vi "Test SSH API.vi"() -> ()   [LabVIEW 2017]
doc: "SSH API Tester."
uses:
  Response Configuration.ctl
  Expected Response String Config.ctl
  Search Start Point.ctl
  Connection Info.ctl
  <vilib>/Utility/config.llb/Write Key (String).vi
  <vilib>/Utility/config.llb/Write Key (I32).vi
  <vilib>/Utility/config.llb/Read Key (String).vi
  <vilib>/Utility/config.llb/Read Key (I32).vi
  SSH.lvlib
  <vilib>/Utility/config.llb/NI_LVConfig.lvlib
panel:
  in  "Load Config":bool
  in  "Save Config":bool
  in  "Write Response Configuration":T1
  in  "password":string
  in  "username":string
  in  "port":i32
  out "Response":string
  in  "Connection Name":string
  in  "host IP":string
  in  "Command":string
  in  "Write Command":bool
  in  "Run as Singleton?":bool
  in  "Show Block Diagram":bool
  in  "Refresh Modules":bool
  out "Active Modules":string[](array[string])
  in  "Stop Module":bool
  in  "Select Module":i32(ring)=-1 caption="Select Module\nTo send Request to" items=["All"=-1]
  in  "Run New Module":bool
  in  "Hide Module Panel":bool
  in  "Show Module Panel":bool
  out "Status":string
  # "This VI tests the API for the Module."
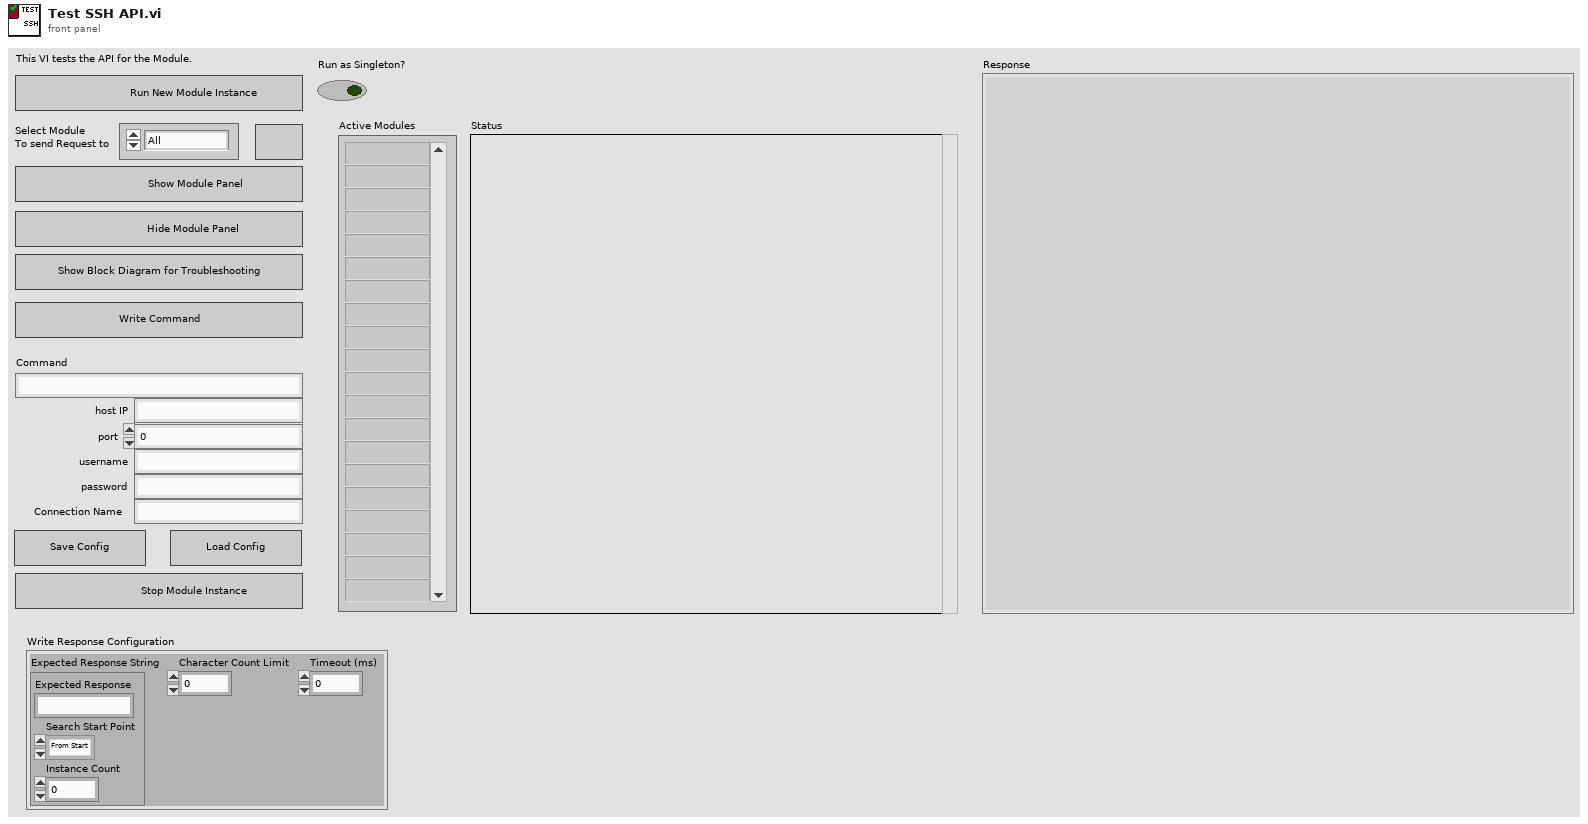
[diagram p1: front panel]
types:
  T1 = typedef "SSH.lvlib/Response Configuration.ctl" = cluster{"Expected Response String":T2, "Character Count Limit":i32, "Timeout (ms)":i32}
  T2 = typedef "SSH.lvlib/Expected Response String Config.ctl" = cluster{"Expected Response":string, "Search Start Point":T3, "Instance Count":i32}
  T3 = typedef "SSH.lvlib/Search Start Point.ctl" = enum16{"From Start", "From End"}
  T4 = typedef "SSH.lvlib/Broadcast Events--cluster.ctl" = cluster{"Module Did Init":refnum<user-event>, "Status Updated":refnum<user-event>, "Error Reported":refnum<user-event>, "Module Did Stop":refnum<user-event>, "Update Module Execution Status":refnum<user-event>}
  T5 = typedef "SSH.lvlib/Connection Info.ctl" = cluster{"host IP":string, "port":i32, "username":string, "password":string, "Connection Name":string}
  T6 = typedef "SSH.lvlib/Write Command (Reply Payload)--cluster.ctl" = cluster{"Write Command_error":errorcluster, "Return String Payload":string}
  T7 = typedef "NI_LVConfig.lvlib/Config Data RefNum.ctl" = refnum<k1>
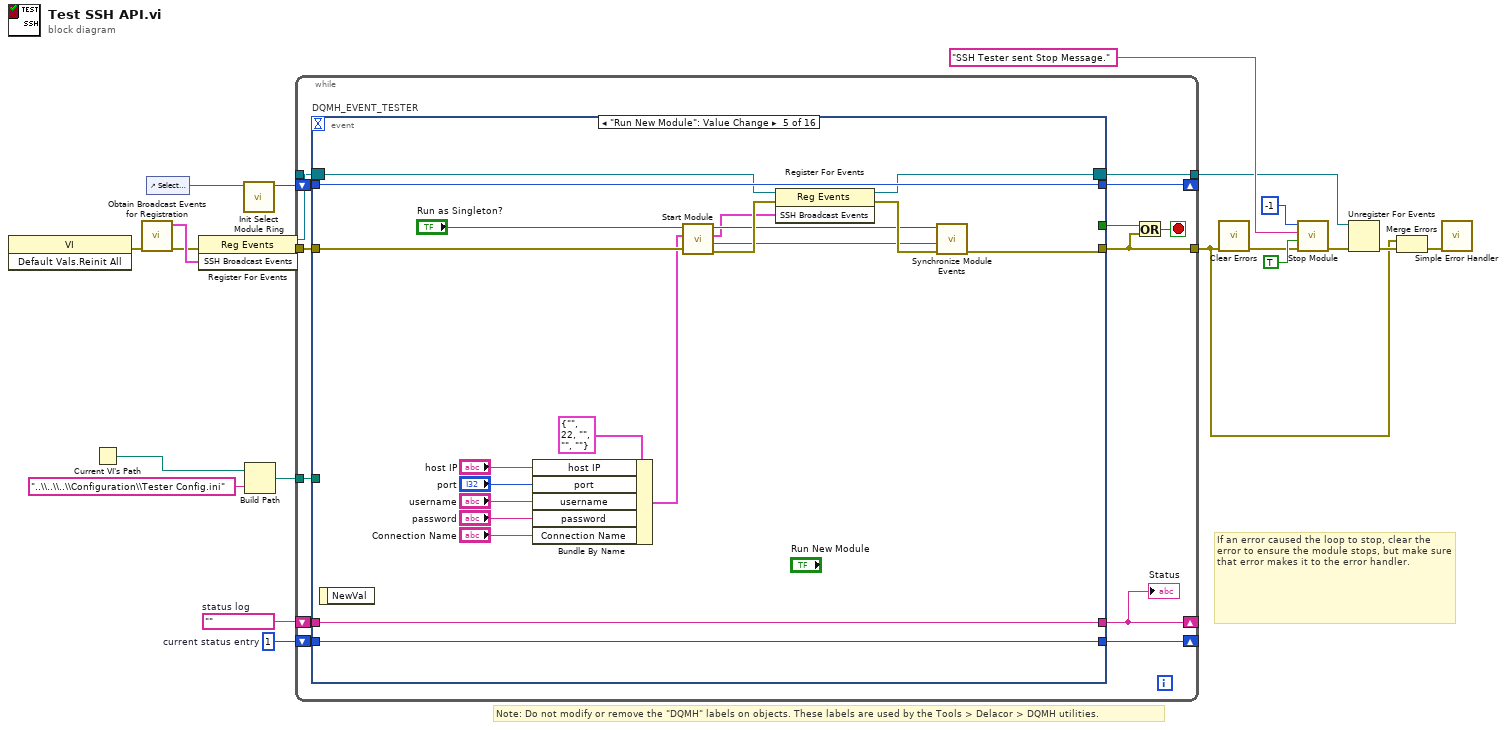
[diagram p0: block diagram]
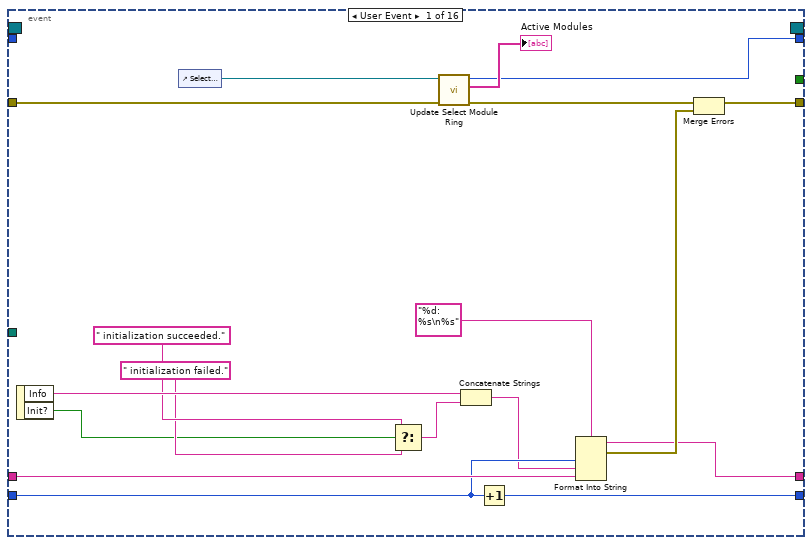
[diagram p2: hidden frame]
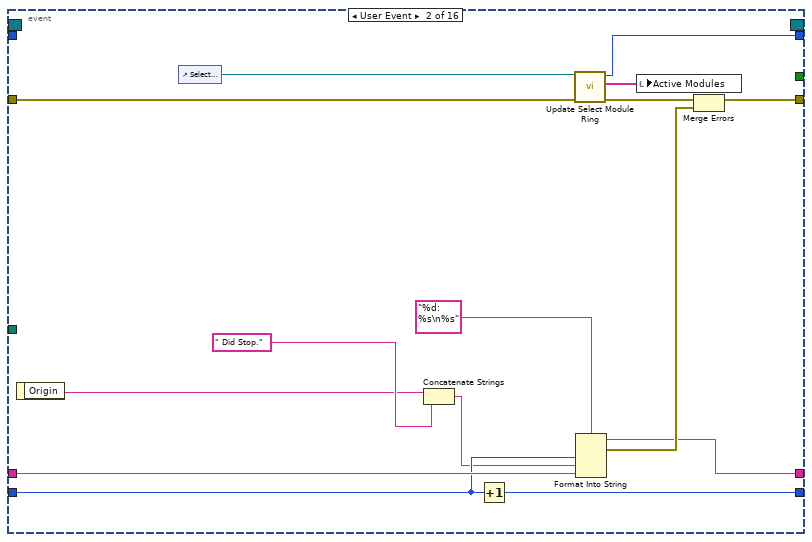
[diagram p3: hidden frame]
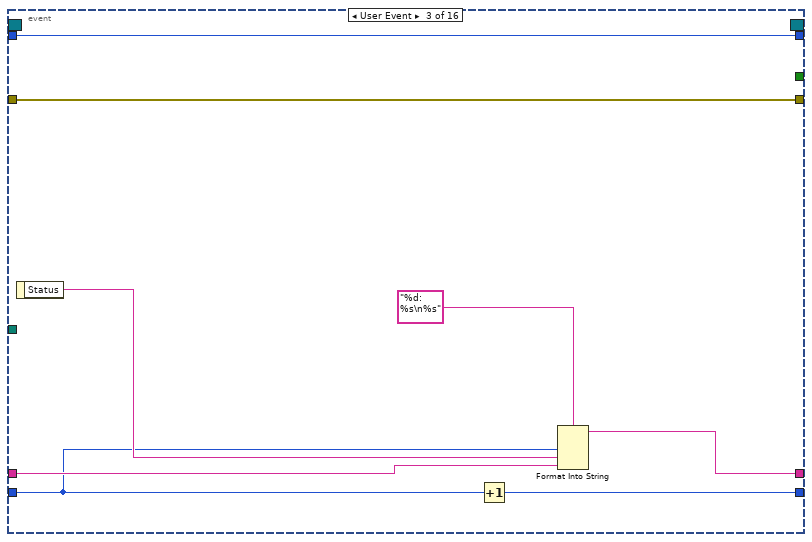
[diagram p4: hidden frame]
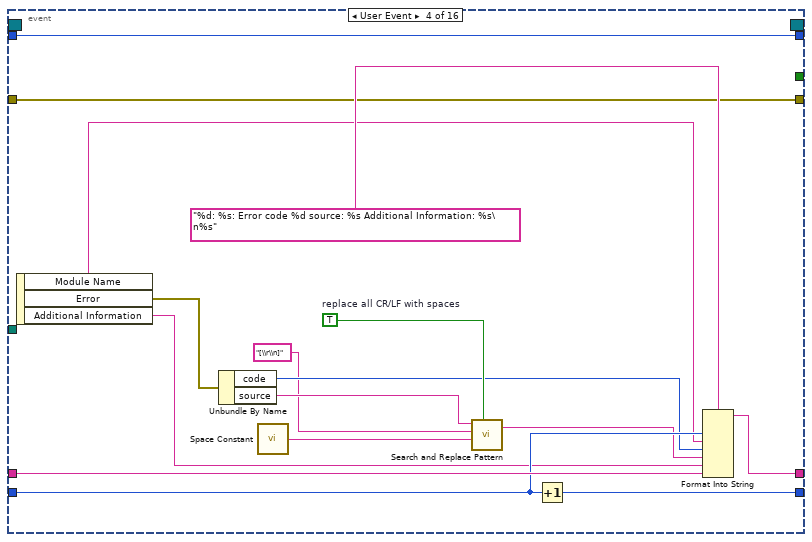
[diagram p5: hidden frame]
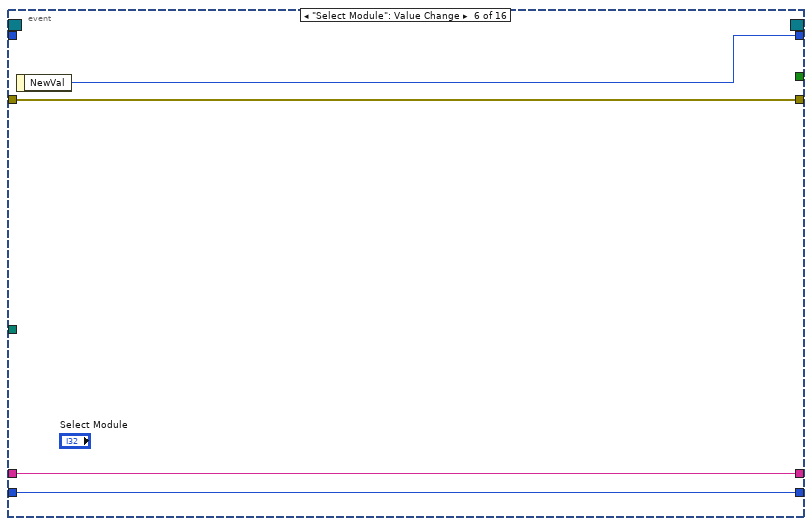
[diagram p6: hidden frame]
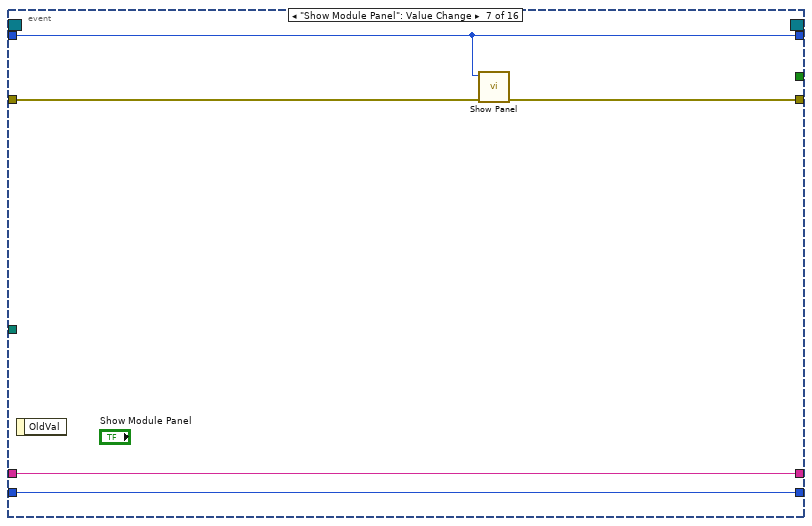
[diagram p7: hidden frame]
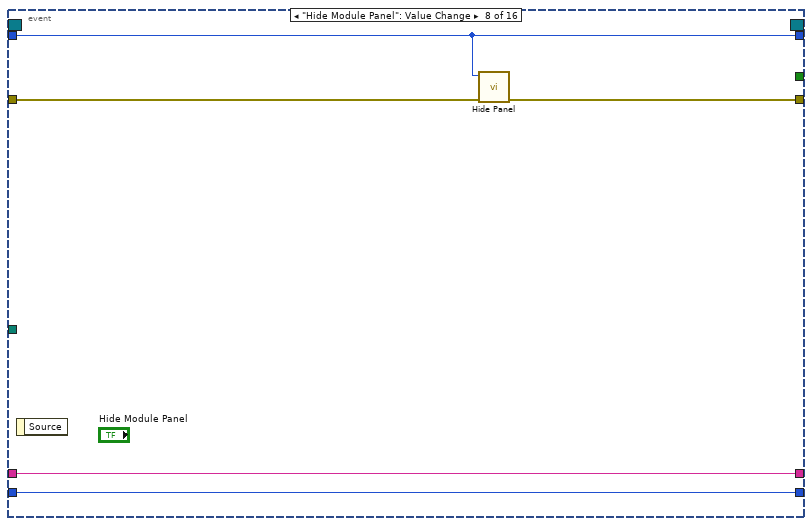
[diagram p8: hidden frame]
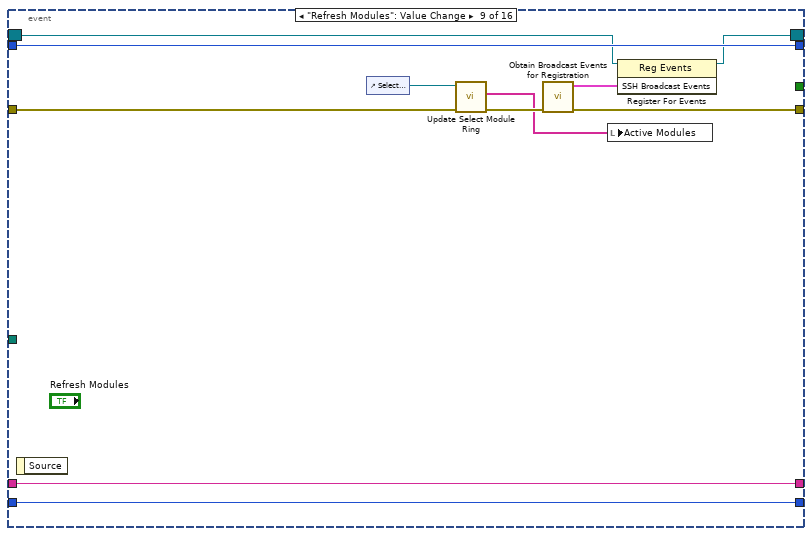
[diagram p9: hidden frame]
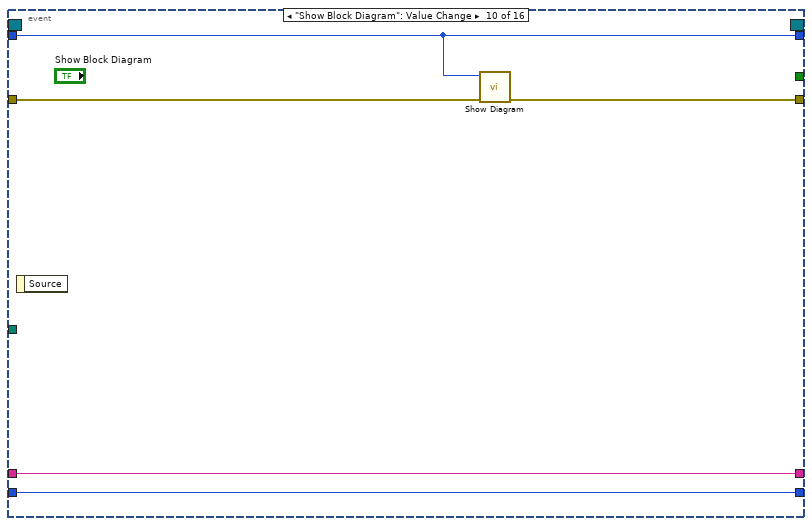
[diagram p10: hidden frame]
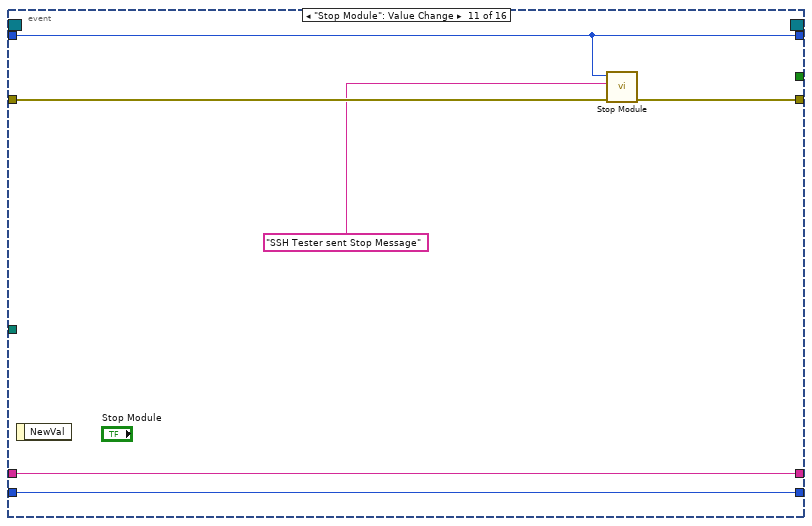
[diagram p11: hidden frame]
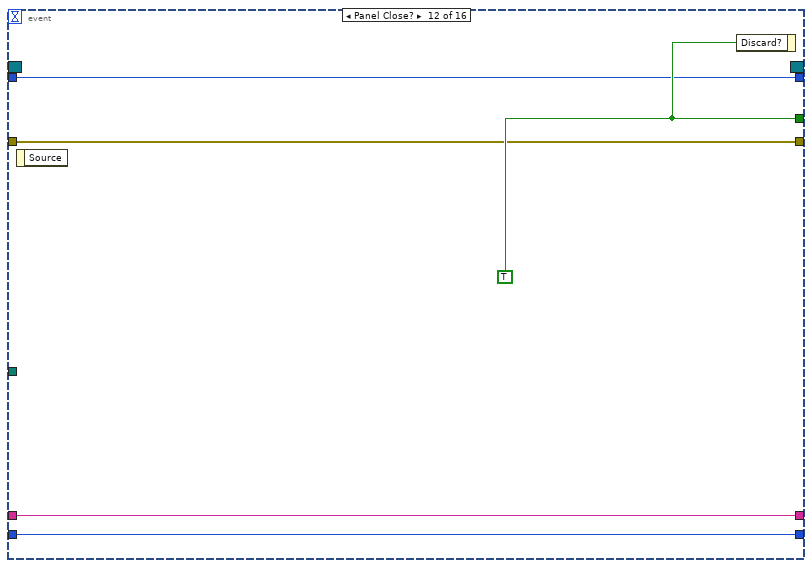
[diagram p12: hidden frame]
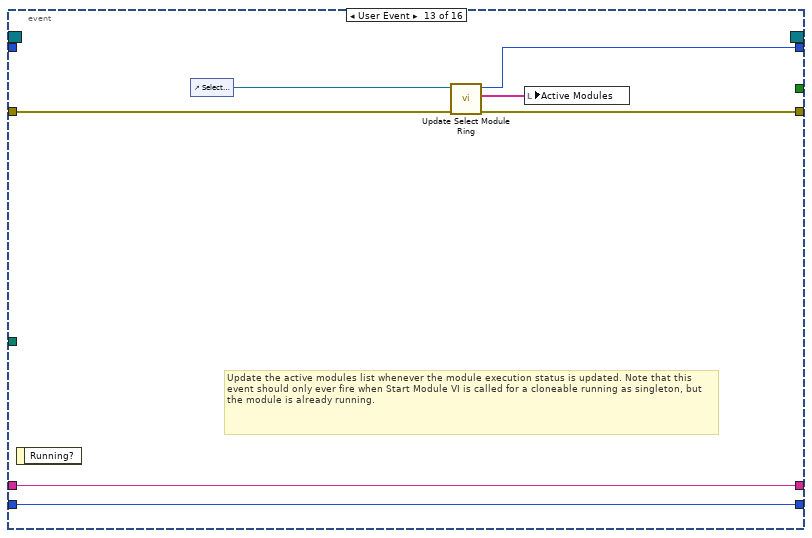
[diagram p13: hidden frame]
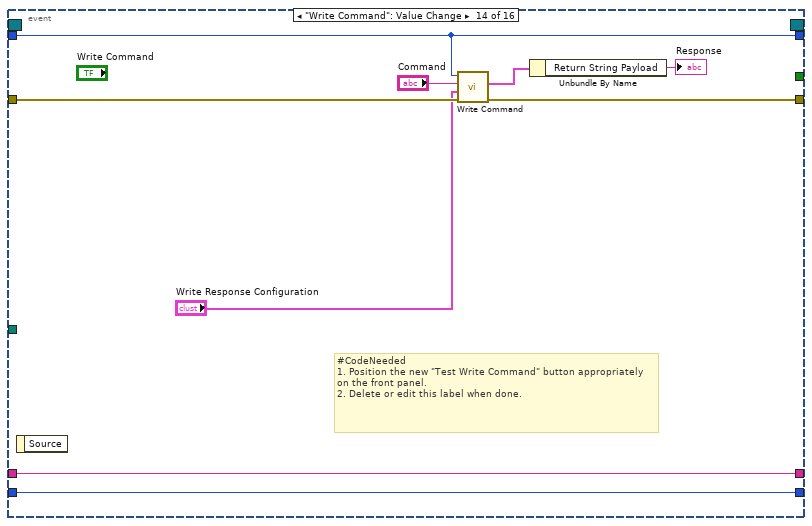
[diagram p14: hidden frame]
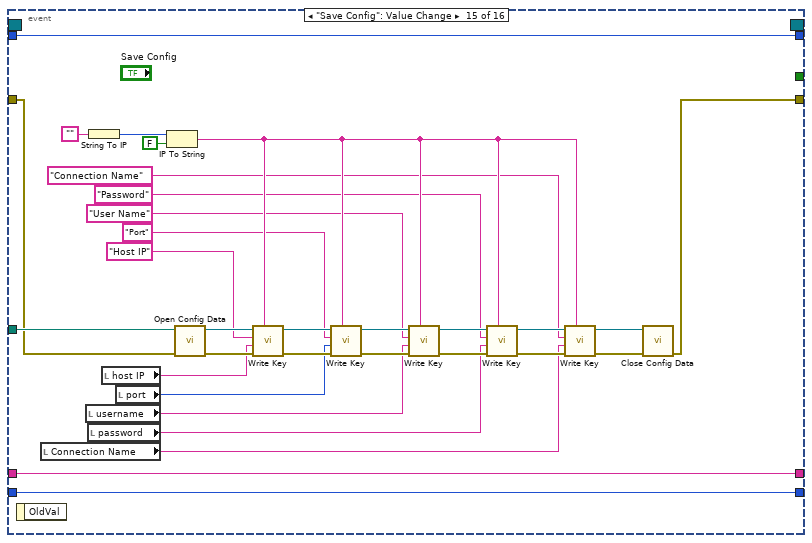
[diagram p15: hidden frame]
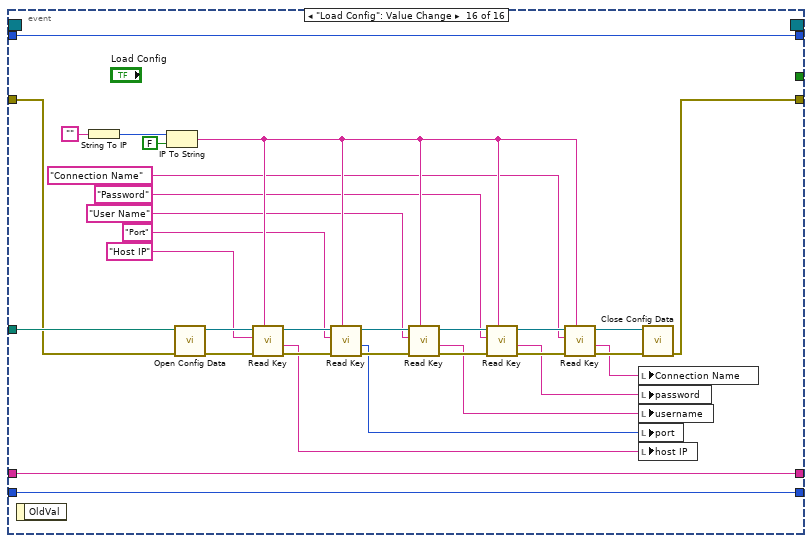
[diagram p16: hidden frame]
diagram:
  w17 = 1  # current status entry
  w18 = ""  # status log
  # "If an error caused the loop to stop, clear the error to ensure the module stops, but make sure that error makes it to the error handler."
  # "Note: Do not modify or remove the \"DQMH\" labels on objects. These labels are used by the Tools > Delacor > DQMH utilities."
  n1 = invoke class="VI" method="Default Vals.Reinit All"() -> (error out=w5:errorcluster)  [unwired: 3 in, 2 out]
  n2 = Current VI's Path() -> (path=w3:path)
  n3 = call "Obtain Broadcast Events for Registration.vi"("error in (no error)"=w5) -> ("error out"=w4:errorcluster, "SSH Broadcast Events"=w14:T4)  [unwired: 9 in]
  n4 = control-ref of="Select Module"() -> (w15:refnum<vi>)
  n5 = register-events(error in=w4, w14) -> (reference out=w21:refnum<event-registration>, error out=w13:errorcluster)  [unwired: 1 in]
  n6 = call "Init Select Module Ring.vi"("Select Module Ring Ref"=w15) -> ("Value for All Modules"=w16:i32)  [unwired: 8 in, 2 out]
  n7 = Build Path(base path=w3, name or relative path="..\\..\\..\\Configuration\\Tester Config.ini") -> (appended path=w1:path)
  n8 = while {
    tunnel: w21 -> [w34]
    tunnel: [w23] -> w6
    tunnel: w13 -> [w32]
    shift-right: [w28] -> _
    shift-left: w18 -> [w30]
    shift-right: [w29] -> _
    shift-left: w17 -> [w31]
    shift-right: [w25] -> _
    shift-left: w16 -> [w26]
    tunnel: [w24] -> w10
    tunnel: w1 -> [w22]
    stop <- w27 stop-if-true
    n9 = event "DQMH_EVENT_TESTER" shown="[4] \"Run New Module\": Value Change" {
      selector: w34 -> [_ _ _ _ w105 _ _ _ w131 _ _ _ _ _ _ _]
      dyn-events: [_ _ _ _ w104 _ _ _ w130 _ _ _ _ _ _ _] -> w24
      timeout: _ -> [_ _ _ _ _ _ _ _ _ _ _ _ _ _ _ _]
      tunnel: [_ _ _ _ _ _ _ _ _ _ _ w152 _ _ _ _] -> w33
      tunnel: [w42 w59 w75 w81 w103 w115 w119 w124 w127 w138 w143 w151 w155 w165 w169 w201] -> w23
      tunnel: w32 -> [w44 w61 w75 w81 w106 w115 w120 w125 w132 w141 w144 w151 w156 w168 w170 w202]
      tunnel: w31 -> [w49 w64 w68 w87 w108 w113 w117 w122 w135 w139 w146 w149 w158 w166 w199 w231]
      tunnel: w30 -> [w50 w65 w71 w89 w109 w114 w118 w123 w136 w140 w147 w150 w159 w167 w200 w232]
      tunnel: [w47 w62 w72 w84 w109 w114 w118 w123 w136 w140 w147 w150 w159 w167 w200 w232] -> w28
      tunnel: [w48 w63 w74 w90 w108 w113 w117 w122 w135 w139 w146 w149 w158 w166 w199 w231] -> w29
      tunnel: w26 -> [_ _ w69 w91 w107 _ w116 w121 w134 w137 w145 w148 _ w164 w198 w230]
      tunnel: [w39 w56 w69 w91 w107 w112 w116 w121 w134 w137 w145 w148 w154 w164 w198 w230] -> w25
      tunnel: w22 -> [_ _ _ _ _ _ _ _ _ _ _ _ _ _ w197 w229]
      event User Event {
        n10 = event-data() -> ("Info"=w46:string, "Init?"=w36:bool)  [unwired: 1 in]
        n11 = control-ref of="Select Module"() -> (w41:refnum<vi>)
        n12 = Select(t=" initialization succeeded.", s=w36, f=" initialization failed.") -> (s? t:f=w35:string)
        n13 = call "Update Select Module Ring.vi"("error in (no error)"=w44, "Select Module Ring Ref"=w41) -> ("error out"=w43:errorcluster, "Active Modules (Array)"=→"Active Modules":string[], "New Module Ring Value"=w39:i32)  [unwired: 7 in]
        n14 = Concatenate Strings(w46, w35) -> (w45:string)
        n15 = Increment(x=w49) -> (x+1=w48:i32)
        n16 = Format Into String(format string="%d: %s\n%s", w49, w45, w50) -> (resulting string=w47:string, error out=w52:errorcluster)  [unwired: 2 in]
        n17 = Merge Errors(w43, w52) -> (w42:errorcluster)
      }
      event User Event {
        n18 = event-data() -> ("Origin"=w54:string)  [unwired: 1 in]
        n19 = control-ref of="Select Module"() -> (w58:refnum<vi>)
        n20 = Concatenate Strings(w54, " Did Stop.") -> (w53:string)
        n21 = Increment(x=w64) -> (x+1=w63:i32)
        n22 = call "Update Select Module Ring.vi"("error in (no error)"=w61, "Select Module Ring Ref"=w58) -> ("error out"=w60:errorcluster, "Active Modules (Array)"=w57:string[], "New Module Ring Value"=w56:i32)  [unwired: 7 in]
        n23 = Format Into String(format string="%d: %s\n%s", w64, w53, w65) -> (resulting string=w62:string, error out=w67:errorcluster)  [unwired: 2 in]
        n24 = local write "Active Modules"(w57) -> ()
        n25 = Merge Errors(w60, w67) -> (w59:errorcluster)
      }
      event User Event {
        n26 = event-data() -> ("Status"=w70:string)  [unwired: 1 in]
        n27 = Increment(x=w68) -> (x+1=w74:i32)
        n28 = Format Into String(format string="%d: %s\n%s", w68, w70, w71) -> (resulting string=w72:string)  [unwired: 2 in, 1 out]
      }
      event User Event {
        w85 = TRUE  # replace all CR/LF with spaces
        n29 = event-data() -> ("Module Name"=w79:string, "Error"=w78:errorcluster, "Additional Information"=w76:string)  [unwired: 1 in]
        n30 = Unbundle By Name(w78) -> ("code"=w80:i32, "source"=w82:string)
        n31 = call <vilib>:"Space Constant.vi"() -> ("String"=w86:string)
        n32 = call <vilib>:"Search and Replace Pattern.vi"("string"=w82, "regular expression (\"\")"="[\\r\\n]" ("regular expression (\"\")"), "replace string (\"\")"=w86, "replace all? (F)"=w85) -> ("result string"=w83:string)  [unwired: 1 in, 1 out]
        n33 = Increment(x=w87) -> (x+1=w90:i32)
        n34 = Format Into String(format string="%d: %s: Error code %d source: %s Additional Information: %s\n%s", w87, w79, w80, w83, w76, w89) -> (resulting string=w84:string)  [unwired: 2 in, 1 out]
      }
      event "Run New Module": Value Change {
        n35 = event-data() -> ()  [unwired: 1 in, 1 out]
        n36 = Bundle By Name(cluster=T5 {"host IP"="", "port"=22, "username"="", "password"="", "Connection Name"=""} ("Connection Info"), "host IP"="host IP", "port"="port", "username"="username", "password"="password", "Connection Name"="Connection Name") -> (w97:T5)
        n37 = call "Start Module.vi"("error in (no error)"=w106, "Connection Info"=w97, "Run as Singleton? (F)"="Run as Singleton?") -> ("error out"=w110:errorcluster, "Wait for Event Sync?"=w101:bool, "SSH Broadcast Events"=w100:T4, "Module ID"=w102:i32)  [unwired: 5 in]
        n38 = register-events(reference=w105, error in=w110, w100) -> (reference out=w104:refnum<event-registration>, error out=w111:errorcluster)
        n39 = call "Synchronize Module Events.vi"("error in (no error)"=w111, "Wait for Event Sync?"=w101, "Module ID"=w102) -> ("error out"=w103:errorcluster)  [unwired: 7 in, 1 out]
      }
      event "Select Module": Value Change {
        n40 = event-data() -> ("NewVal"=w112:i32)  [unwired: 1 in]
      }
      event "Show Module Panel": Value Change {
        n41 = event-data() -> ()  [unwired: 1 in, 1 out]
        n42 = call "Show Panel.vi"("error in (no error)"=w120, "Module ID"=w116) -> ("error out"=w119:errorcluster)  [unwired: 9 in]
      }
      event "Hide Module Panel": Value Change {
        n43 = event-data() -> ()  [unwired: 1 in, 1 out]
        n44 = call "Hide Panel.vi"("error in (no error)"=w125, "Module ID"=w121) -> ("error out"=w124:errorcluster)  [unwired: 9 in]
      }
      event "Refresh Modules": Value Change {
        n45 = event-data() -> ()  [unwired: 1 in, 1 out]
        n46 = control-ref of="Select Module"() -> (w133:refnum<vi>)
        n47 = call "Update Select Module Ring.vi"("error in (no error)"=w132, "Select Module Ring Ref"=w133) -> ("error out"=w128:errorcluster, "Active Modules (Array)"=w126:string[])  [unwired: 7 in, 1 out]
        n48 = call "Obtain Broadcast Events for Registration.vi"("error in (no error)"=w128) -> ("error out"=w127:errorcluster, "SSH Broadcast Events"=w129:T4)  [unwired: 9 in]
        n49 = local write "Active Modules"(w126) -> ()
        n50 = register-events(reference=w131, w129) -> (reference out=w130:refnum<event-registration>)  [unwired: 1 in, 1 out]
      }
      event "Show Block Diagram": Value Change {
        n51 = event-data() -> ()  [unwired: 1 in, 1 out]
        n52 = call "Show Diagram.vi"("error in (no error)"=w141, "Module ID"=w137) -> ("error out"=w138:errorcluster)  [unwired: 9 in]
      }
      event "Stop Module": Value Change {
        n53 = event-data() -> ()  [unwired: 1 in, 1 out]
        n54 = call "Stop Module.vi"("error in (no error)"=w144, "Origin"="SSH Tester sent Stop Message", "Module ID"=w145) -> ("error out"=w143:errorcluster)  [unwired: 8 in]
      }
      event Panel Close? {
        w152 = TRUE ("Discard?")
        n55 = event-data() -> ()  [unwired: 1 in, 1 out]
        n56 = event-data("Discard?"=w152) -> ()  [unwired: 1 in, 1 out]
      }
      event User Event {
        # "Update the active modules list whenever the module execution status is updated. Note that this event should only ever fire when Start Module VI is called for a cloneable running as singleton, but the module is already running."
        n57 = event-data() -> ()  [unwired: 1 in, 1 out]
        n58 = control-ref of="Select Module"() -> (w157:refnum<vi>)
        n59 = call "Update Select Module Ring.vi"("error in (no error)"=w156, "Select Module Ring Ref"=w157) -> ("error out"=w155:errorcluster, "Active Modules (Array)"=w153:string[], "New Module Ring Value"=w154:i32)  [unwired: 7 in]
        n60 = local write "Active Modules"(w153) -> ()
      }
      event "Write Command": Value Change {
        # "#CodeNeeded\n1. Position the new \"Test Write Command\" button appropriately on the front panel.\n2. Delete or edit this label when done."
        n61 = event-data() -> ()  [unwired: 1 in, 1 out]
        n62 = call "Write Command.vi"("error in (no error)"=w168, "Response Configuration"="Write Response Configuration", "Command"="Command", "Module ID"=w164) -> ("error out"=w165:errorcluster, "Reply Payload"=w162:T6)  [unwired: 5 in, 1 out]
        n63 = Unbundle By Name(w162) -> ("Return String Payload"=→"Response":string)
      }
      event "Save Config": Value Change {
        n64 = event-data() -> ()  [unwired: 1 in, 1 out]
        n65 = local read "Connection Name"() -> (w176:string)
        n66 = local read "username"() -> (w178:string)
        n67 = local read "password"() -> (w177:string)
        n68 = String To IP(1:"") -> (0:w194:u32)
        n69 = local read "host IP"() -> (w180:string)
        n70 = local read "port"() -> (w179:i32)
        n71 = IP To String(1:FALSE ("dot notation? (F)"), 2:w194) -> (0:w181:string)
        n72 = call <vilib>:"Open Config Data.vi"("error in (no error)"=w170, "configuration file path"=w197) -> ("error out"=w192:errorcluster, "refnum"=w193:T7)  [unwired: 7 in, 1 out]
        n73 = call-poly <vilib>:"Write Key.vi"("section"=w181, "error in (no error)"=w192, "value"=w180, "key"="Host IP", "refnum"=w193) -> ("error out"=w190:errorcluster, "refnum out"=w191:T7)  [unwired: 4 in, 1 out]
        n74 = call-poly <vilib>:"Write Key.vi"("section"=w181, "error in (no error)"=w190, "value"=w179, "key"="Port", "refnum"=w191) -> ("error out"=w188:errorcluster, "refnum out"=w189:T7)  [unwired: 4 in, 1 out]
        n75 = call-poly <vilib>:"Write Key.vi"("section"=w181, "error in (no error)"=w188, "value"=w178, "key"="User Name", "refnum"=w189) -> ("error out"=w186:errorcluster, "refnum out"=w187:T7)  [unwired: 4 in, 1 out]
        n76 = call-poly <vilib>:"Write Key.vi"("section"=w181, "error in (no error)"=w186, "value"=w177, "key"="Password", "refnum"=w187) -> ("error out"=w184:errorcluster, "refnum out"=w185:T7)  [unwired: 4 in, 1 out]
        n77 = call-poly <vilib>:"Write Key.vi"("section"=w181, "error in (no error)"=w184, "value"=w176, "key"="Connection Name", "refnum"=w185) -> ("error out"=w182:errorcluster, "refnum out"=w183:T7)  [unwired: 4 in, 1 out]
        n78 = call <vilib>:"Close Config Data.vi"("error in (no error)"=w182, "refnum"=w183) -> ("error out"=w169:errorcluster)  [unwired: 8 in, 1 out]
      }
      event "Load Config": Value Change {
        n79 = event-data() -> ()  [unwired: 1 in, 1 out]
        n80 = String To IP(1:"") -> (0:w226:u32)
        n81 = IP To String(1:FALSE ("dot notation? (F)"), 2:w226) -> (0:w213:string)
        n82 = call <vilib>:"Open Config Data.vi"("error in (no error)"=w202, "configuration file path"=w229) -> ("error out"=w224:errorcluster, "refnum"=w225:T7)  [unwired: 7 in, 1 out]
        n83 = call-poly <vilib>:"Read Key.vi"("section"=w213, "error in (no error)"=w224, "key"="Host IP", "refnum"=w225) -> ("error out"=w222:errorcluster, "value"=w203:string, "refnum out"=w223:T7)  [unwired: 4 in, 1 out]
        n84 = call-poly <vilib>:"Read Key.vi"("section"=w213, "error in (no error)"=w222, "key"="Port", "refnum"=w223) -> ("error out"=w220:errorcluster, "value"=w204:i32, "refnum out"=w221:T7)  [unwired: 4 in, 1 out]
        n85 = call-poly <vilib>:"Read Key.vi"("section"=w213, "error in (no error)"=w220, "key"="User Name", "refnum"=w221) -> ("error out"=w218:errorcluster, "value"=w205:string, "refnum out"=w219:T7)  [unwired: 4 in, 1 out]
        n86 = call-poly <vilib>:"Read Key.vi"("section"=w213, "error in (no error)"=w218, "key"="Password", "refnum"=w219) -> ("error out"=w216:errorcluster, "value"=w206:string, "refnum out"=w217:T7)  [unwired: 4 in, 1 out]
        n87 = call-poly <vilib>:"Read Key.vi"("section"=w213, "error in (no error)"=w216, "key"="Connection Name", "refnum"=w217) -> ("error out"=w214:errorcluster, "value"=w207:string, "refnum out"=w215:T7)  [unwired: 4 in, 1 out]
        n88 = local write "Connection Name"(w207) -> ()
        n89 = local write "password"(w206) -> ()
        n90 = local write "username"(w205) -> ()
        n91 = local write "port"(w204) -> ()
        n92 = local write "host IP"(w203) -> ()
        n93 = call <vilib>:"Close Config Data.vi"("error in (no error)"=w214, "refnum"=w215) -> ("error out"=w201:errorcluster)  [unwired: 8 in, 1 out]
      }
    }
    "Status" <- w28
    n94 = Or(x=w33, y=w23) -> (x .or. y?=w27:bool)
  }
  n95 = call <vilib>:"Clear Errors.vi"("error in (no error)"=w6) -> ("error out"=w8:errorcluster)  [unwired: 5 in, 1 out]
  n96 = call "Stop Module.vi"("error in (no error)"=w8, "Wait for Module to stop? (F)"=TRUE ("Wait for Module to stop?"), "Origin"="SSH Tester sent Stop Message.", "Module ID"=-1 ("Stop all")) -> ("error out"=w19:errorcluster)  [unwired: 7 in]
  n97 = Unregister For Events(event registration refnum=w10, error in=w19) -> (error out=w20:errorcluster)
  n98 = Merge Errors(w6, w20) -> (w7:errorcluster)
  n99 = call <vilib>:"Simple Error Handler.vi"("error in (no error)"=w7) -> ()  [unwired: 4 in, 5 out]
